vi "CLC_Single_Channel_COM_CMD.vi"(7 "Channel params":T1={"Mode"=1, "Polarity"=1, "CH_ON/OFF"=1, "Channel"=0, "Gain"=0, "Phase"=0} {"CH_ON/OFF" items=["ON", "OFF"]; "Polarity" items=["H", "V"]; "Mode" items=["Tx"=1, "Rx"=2]}, 8 "error in":errorcluster, 11 "TCPIPin":T2={"address"="192.168.100.111", "remote port or service name"=5025, "timeout ms (60000)"=10000}) -> (0 "error out":errorcluster, 1 "OK?":bool, 3 "TCPIPout":T2={"address"="192.168.100.111", "remote port or service name"=5025, "timeout ms (60000)"=10000})   [LabVIEW 2023]
panel:
  out "cmd":string
  out "data out":string
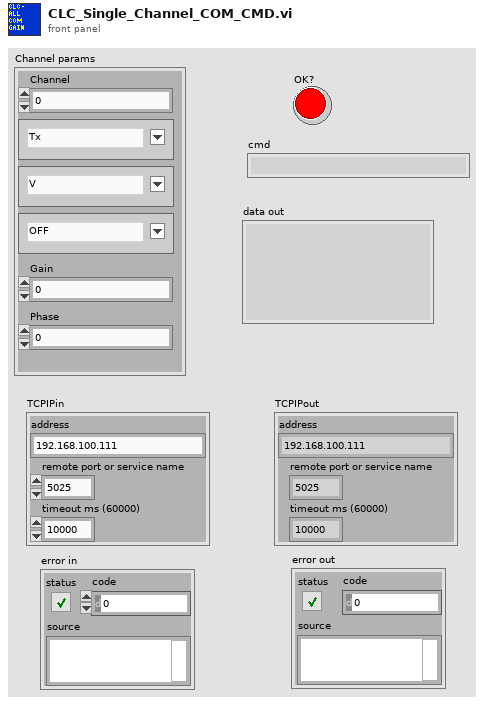
[diagram p1: front panel]
types:
  T1 = cluster{"Mode":u16, "Polarity":u16, "CH_ON/OFF":u16, "Channel":i32, "Gain":i32, "Phase":i32}
  T2 = cluster{"address":string, "remote port or service name":u16, "timeout ms (60000)":i32}
  T3 = enum16{"Standard", "Buffered", "CRLF", "Immediate"}
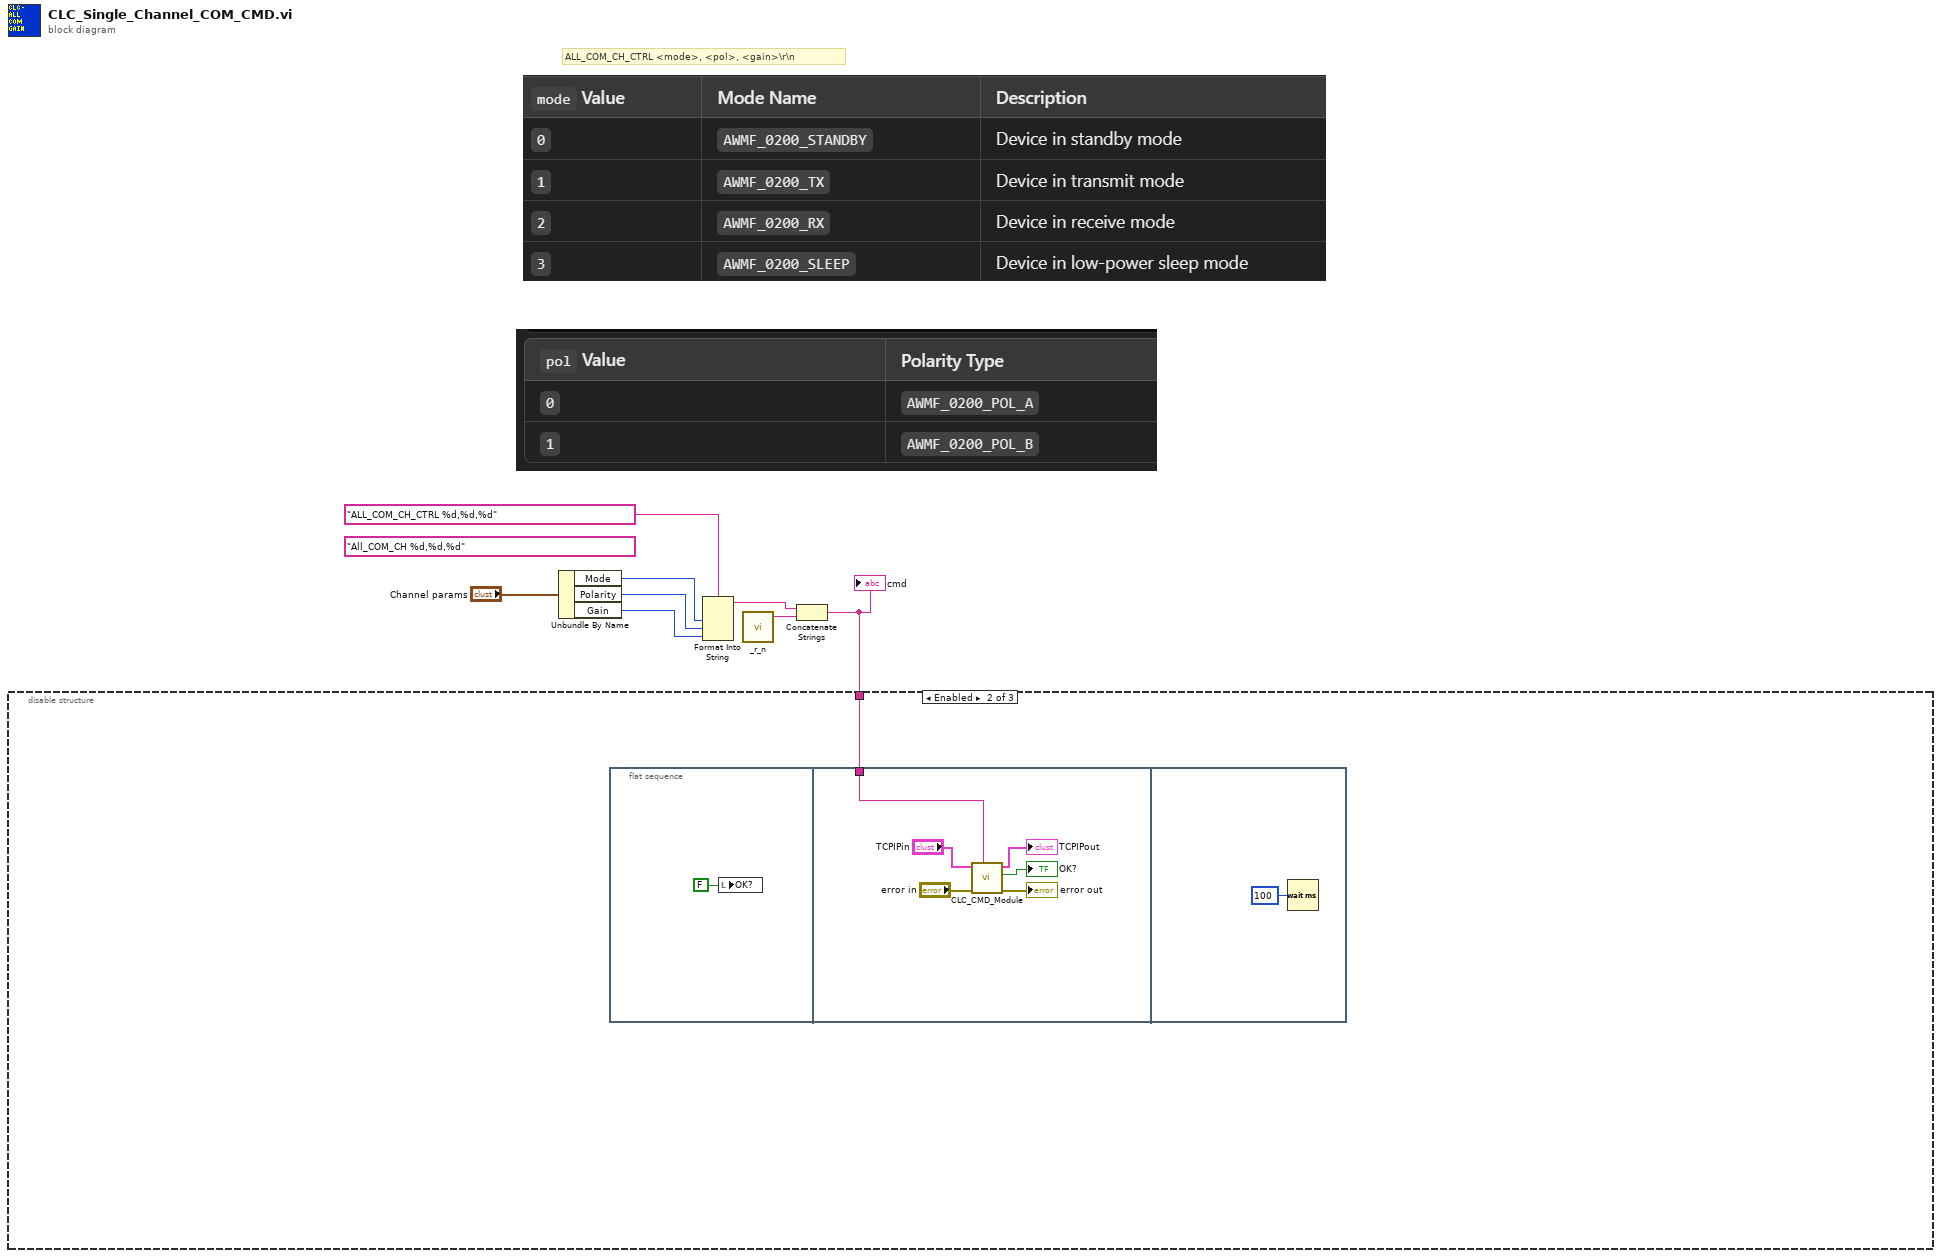
[diagram p0: block diagram]
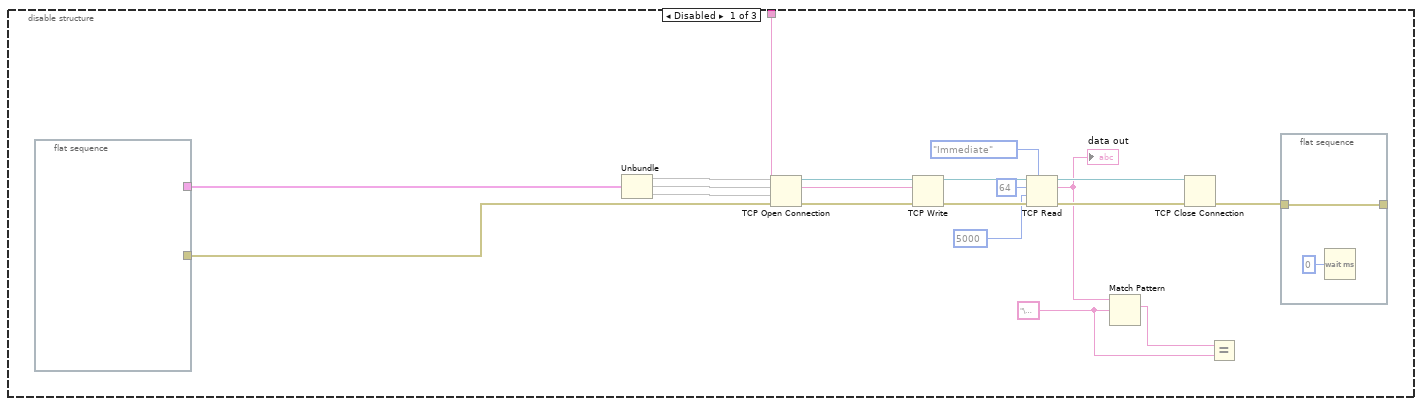
[diagram p2: hidden frame]
diagram:
  (unwired) "All_COM_CH %d,%d,%d" ("data in")
  # "ALL_COM_CH_CTRL <mode>, <pol>, <gain>\\r\\n"
  n1 = Unbundle By Name("Channel params") -> ("Mode"=w4:u16, "Polarity"=w3:u16, "Gain"=w2:i32)
  n2 = Format Into String(format string="ALL_COM_CH_CTRL %d,%d,%d" ("data in"), w4, w3, w2) -> (resulting string=w7:string)  [unwired: 2 in, 1 out]
  n3 = call "_r_n.vi"() -> ("command"=w6:string)  [unwired: 5 in]
  n4 = Concatenate Strings(w7, w6) -> (w8:string)
  "cmd" <- w8
  n5 = disable-structure shown="Enabled" {
    disable-tunnel: w8 -> [w23 w30 _]
    frame Disabled {
      w10 = "\u0000" ("string")
      n6 = flat-sequence {
        tunnel: [_] -> w27
        tunnel: [_] -> w26
        frame #0 {
        }
      }
      n7 = Unbundle(w27) -> ("address"=w22, "remote port or service name"=w21, "timeout ms (60000)"=w20)
      n8 = TCP Open Connection(address=w22, remote port or service name=w21, timeout ms (60000)=w20, error in (no error)=w26) -> (connection ID=w25:refnum<k5>, error out=w24:errorcluster)  [unwired: 1 in]
      n9 = TCP Write(connection ID=w25, data in=w23, error in (no error)=w24) -> (connection ID out=w18:refnum<k5>, error out=w19:errorcluster)  [unwired: 1 in, 1 out]
      n10 = TCP Read(connection ID=w18, bytes to read=64, error in (no error)=w19, 7:T3."Immediate" ("mode (standard)"), 9:5000 ("timeout ms (25000)")) -> (connection ID out=w17:refnum<k5>, data out=w12:string, error out=w16:errorcluster)
      "data out" <- w12
      n11 = Match Pattern(string=w12, regular expression=w10) -> (match substring=w11:string)  [unwired: 1 in, 3 out]
      n12 = TCP Close Connection(connection ID=w17, error in (no error)=w16) -> (error out=w9:errorcluster)  [unwired: 1 in, 1 out]
      n13 = Equal?(x=w11, y=w10) -> ()  [unwired: 1 out]
      n14 = flat-sequence {
        tunnel: w9 -> [w29]
        tunnel: [w29] -> _
        frame #0 {
          n15 = Wait (ms)(milliseconds to wait=u32 0) -> ()  [unwired: 1 out]
        }
      }
    }
    frame Enabled {
      n16 = flat-sequence {
        tunnel: w30 -> [w35]
        frame #0 {
          n17 = local write "OK?"(FALSE ("OK?")) -> ()
        }
        frame #1 {
          n18 = call "CLC_CMD_Module.vi"("CMD in"=w35, "error in"="error in", "TCPIPin"="TCPIPin") -> ("error out"=→"error out":errorcluster, "OK?"=→"OK?":bool, "TCPIPout"=→"TCPIPout":T2)  [unwired: 5 in, 1 out]
        }
        frame #2 {
          n19 = Wait (ms)(milliseconds to wait=u32 100) -> ()  [unwired: 1 out]
        }
      }
    }
    frame Disabled {
    }
  }
